vi "BorderInterpolate.vi"(6 "BorderTypes":T1=4 items=["BORDER_CONSTANT"=0, "BORDER_REPLICATE"=1, "BORDER_REFLECT"=2, "BORDER_WRAP"=3, "BORDER_REFLECT_101"=4, "BORDER_TRANSPARENT"=5, "BORDER_ISOLATED"=16], 8 "error in":errorcluster, 10 "len":i32, 11 "p":i32) -> (0 "error out":errorcluster, 3 "Value":i32)   [LabVIEW 2020, in "OpenLvVision_OpenCv.lvlib"]
doc: "Computes the source location of an extrapolated pixel."
uses:
  OpenLvVision_OpenCv.lvlib
  TypeDef/BorderTypes.ctl
  Dlls/OlvOpenCvWrapper.dll
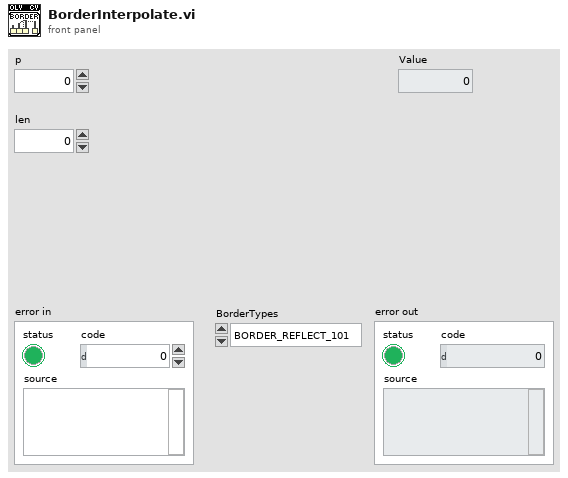
[diagram p1: front panel]
types:
  T1 = typedef "OpenLvVision_OpenCv.lvlib/BorderTypes.ctl" = i32
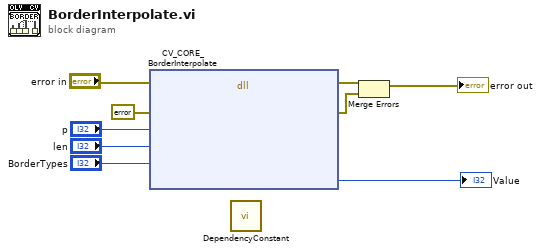
[diagram p0: block diagram]
diagram:
  n1 = dll-call lib="C:/Users/lukas/Downloads/OpenLvVision_OpenCv/SourceCode/LabView/OpenLvVision_OpenCv/Dlls/OlvOpenCvWrapper.dll" fn="CV_CORE_BorderInterpolate"(error in="error in", "Error"=errorcluster {"status"=FALSE, "code"=0, "source"=""} ("error constant"), "p"="p", "len"="len", "borderType"="BorderTypes") -> (error out=w8:errorcluster, "Error"=w4:errorcluster, "value"=→"Value":i32)  [unwired: 7 in, 1 out]
  n2 = call "DependencyConstant.vi"() -> ()  [unwired: 12 in]
  n3 = Merge Errors(w8, w4) -> (→"error out":errorcluster)
